vi "ATF-Config Array Value ref.vi"(9 "Value":variant, 11 "Array in":refnum<vi>) -> (0 "error out":errorcluster)   [LabVIEW 2022 SP3]
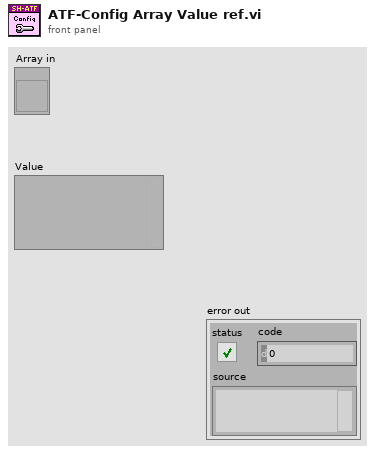
[diagram p1: front panel]
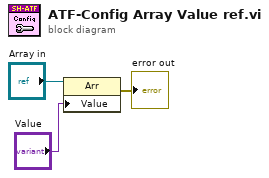
[diagram p0: block diagram]
diagram:
  n1 = property class="Arr"(reference="Array in", "Value"="Value") -> (error out=→"error out":errorcluster)  [unwired: 1 in, 1 out]
